vi "Size (Greyscale).vi"(8 "error in (no error)":errorcluster, 11 "Greyscale Image in":T1) -> (0 "error out":errorcluster, 2 "Image Size":T2, 3 "Greyscale Image":T1)   [LabVIEW 2020, in "image.lvlib"]
doc: "Get the Size of the Image."
uses:
  image.lvlib
  Greyscale Image.ctl
  common/Image Size (Integer).ctl
  69a1505b-b287-44ed-9ef9-f10ed7b260f4.vi
  common/common.lvlib
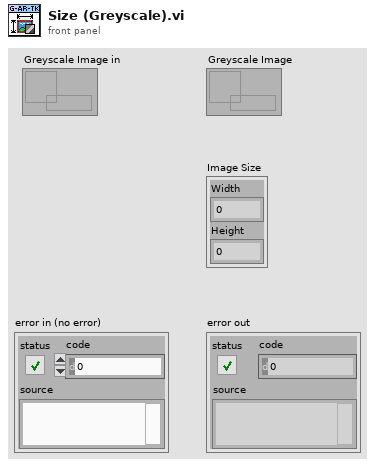
[diagram p1: front panel]
types:
  T1 = typedef "image.lvlib/Greyscale Image.ctl" = refnum<data-value>
  T2 = typedef "common.lvlib/Image Size (Integer).ctl" = cluster{"Width":u16, "Height":u16}
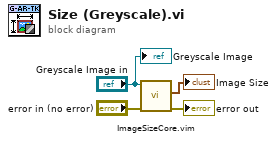
[diagram p0: block diagram]
diagram:
  n1 = call "ImageSizeCore.vim"("error in (no error)"="error in (no error)", "Image"="Greyscale Image in") -> ("error out"=→"error out":errorcluster, "Image Size"=→"Image Size":T2)  [unwired: 8 in]
  "Greyscale Image" <- "Greyscale Image in"
